vi "Multi-Carrier Modulation.vi"() -> ()   [LabVIEW 2018]
uses:
  <vilib>/measure/maspectr.llb/FFT Spectrum (Real-Im) for 1 Chan (CDB).vi
  <vilib>/measure/NI_MAPro.lvlib
panel:
  out "FFT Complex":cluster{"f0":dbl, "df":dbl, "real part":dbl[]}(graph)
  out "FFT Real":cluster{"f0":dbl, "df":dbl, "real part":dbl[]}(graph)
  in  "QAM Comparison":enum16{"MT Modulate", "Homebrew"}(ring)
  out "Waveform Chart":dbl[][](graph)
  out "Minimum Sampling Rate":dbl
  in  "Lowest f":dbl=1.0 format="%0.2p"
  in  "DataLen":i32=512
  in  "QAM Complexity":T1(ring)
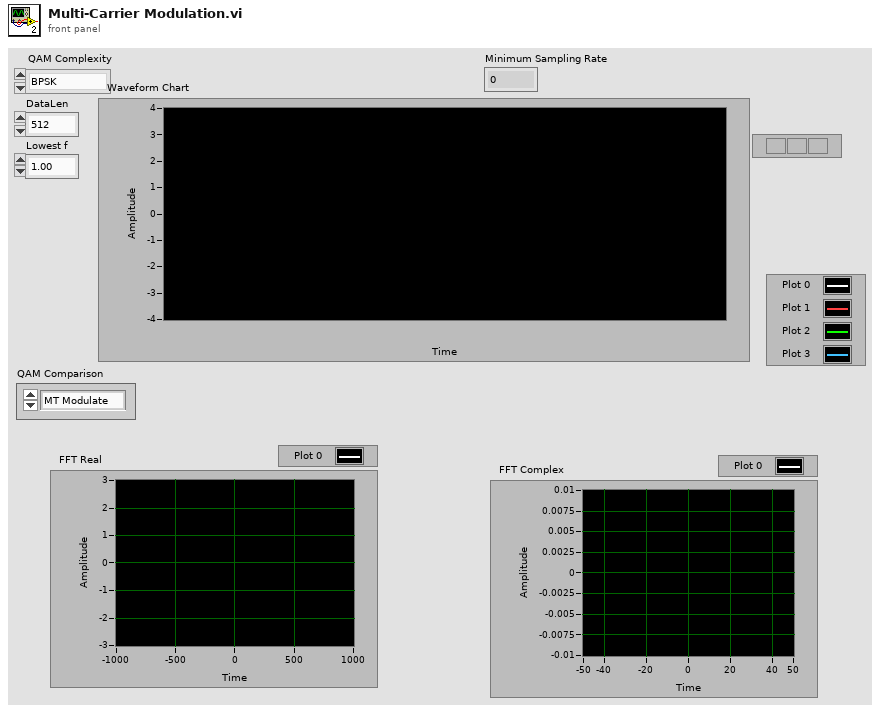
[diagram p1: front panel]
types:
  T1 = enum16{"BPSK", "QPSK", "16-QAM", "64-QAM", "256-QAM"}
  T2 = cluster{"f0":dbl, "df":dbl, "imaginary part":dbl[]}
  T3 = typedef "NI_Matrix.lvlib/ComplexMatrix.ctl" = cdb[][]
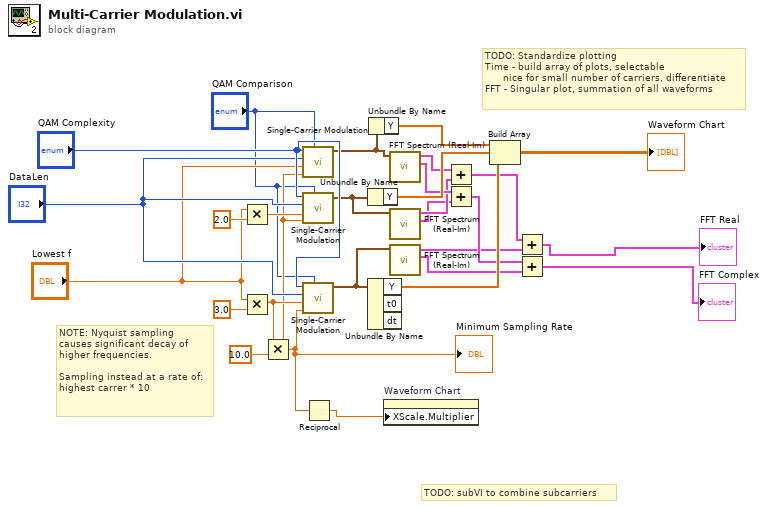
[diagram p0: block diagram]
diagram:
  # "TODO: subVI to combine subcarriers"
  # "TODO: Standardize plotting\nTime - build array of plots, selectable\n      nice for small number of carriers, differentiate\nFFT - Singular plot, summation of all waveforms"
  # "NOTE: Nyquist sampling\ncauses significant decay of \nhigher frequencies. \n\nSampling instead at a rate of:\nhighest carrer * 10"
  n1 = Multiply(x="Lowest f", y=2.0) -> (x*y=w28:dbl)
  n2 = Multiply(x="Lowest f", y=3.0) -> (x*y=w22:dbl)
  n3 = Multiply(x=w22, y=10.0) -> (x*y=w15:dbl)
  "Minimum Sampling Rate" <- w15
  n4 = call "Single-Carrier Modulation.vi"("QAM Comparison"="QAM Comparison", "Sampling Rate"=w15, "frequency"="Lowest f", "DataLen"="DataLen", "QAM Complexity"="QAM Complexity") -> ("waveform"=w13:waveform(cdb))  [unwired: 5 in, 1 out]
  n5 = call "Single-Carrier Modulation.vi"("QAM Comparison"="QAM Comparison", "Sampling Rate"=w15, "frequency"=w28, "DataLen"="DataLen", "QAM Complexity"="QAM Complexity") -> ("waveform"=w12:waveform(cdb))  [unwired: 5 in, 1 out]
  n6 = call "Single-Carrier Modulation.vi"("QAM Comparison"="QAM Comparison", "Sampling Rate"=w15, "frequency"=w22, "DataLen"="DataLen", "QAM Complexity"="QAM Complexity") -> ("waveform"=w11:waveform(cdb))  [unwired: 5 in, 1 out]
  n7 = Reciprocal(x=w15) -> (1/x=w16:dbl)
  n8 = Unbundle By Name(w12) -> ("Y"=w19:cdb[])
  n9 = Unbundle By Name(w11) -> ("Y"=w18:cdb[])  [unwired: 2 out]
  n10 = Unbundle By Name(w13) -> ("Y"=w20:cdb[])
  n11 = property on="Waveform Chart" class="WFChart (strict)"("XScale.Multiplier"=w16) -> ()  [unwired: 2 in, 2 out]
  n12 = call-poly <vilib>:"FFT Spectrum (Real-Im).vi"("time signal"=w13) -> ("imaginary part"=w9:T2, "real part"=w10:cluster{"f0":dbl, "df":dbl, "real part":dbl[]})  [unwired: 6 in, 3 out]
  n13 = call-poly <vilib>:"FFT Spectrum (Real-Im).vi"("time signal"=w12) -> ("imaginary part"=w7:T2, "real part"=w8:cluster{"f0":dbl, "df":dbl, "real part":dbl[]})  [unwired: 6 in, 3 out]
  n14 = call-poly <vilib>:"FFT Spectrum (Real-Im).vi"("time signal"=w11) -> ("imaginary part"=w3:T2, "real part"=w4:cluster{"f0":dbl, "df":dbl, "real part":dbl[]})  [unwired: 6 in, 3 out]
  n15 = Add(x=w10, y=w8) -> (x+y=w6:cluster{"f0":dbl, "df":dbl, "real part":dbl[]})
  n16 = Add(x=w9, y=w7) -> (x+y=w5:T2)
  n17 = Build Array(w20, w19, w18) -> (→"Waveform Chart":T3)
  n18 = Add(x=w6, y=w4) -> (x+y=→"FFT Real":cluster{"f0":dbl, "df":dbl, "real part":dbl[]})
  n19 = Add(x=w5, y=w3) -> (x+y=→"FFT Complex":T2)
